vi "meTEC_Read_Firmware Indentification String.vi"(8 "error in (no error)":errorcluster, 9 "TEC Configuration_IN":T1={"VISA resource name"="", "Device Address"=2}, 11 "Sequence No.":u16=5546) -> (0 "error out":errorcluster, 1 "TEC Configuration_OUT":T1={"VISA resource name"="", "Device Address"=2}, 3 "Firmware Identification String":string)   [LabVIEW 2019]
uses:
  TypeDefs/meTEC_Configuration.ctl
panel:
  # "--- Inputs ---"
  # "--- Outputs ---"
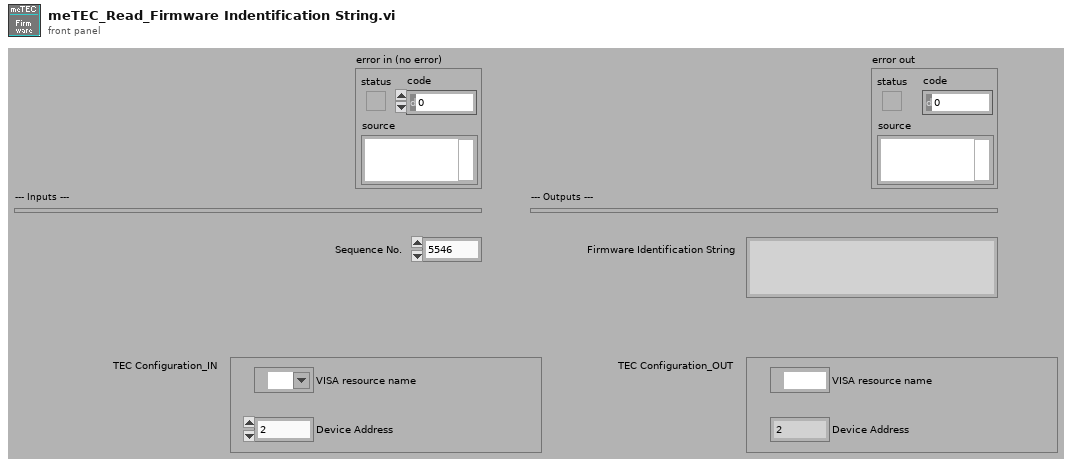
[diagram p1: front panel]
types:
  T1 = typedef "meTEC_Configuration.ctl" = cluster{"VISA resource name":refnum<visa-resource-name>, "Device Address":u16}
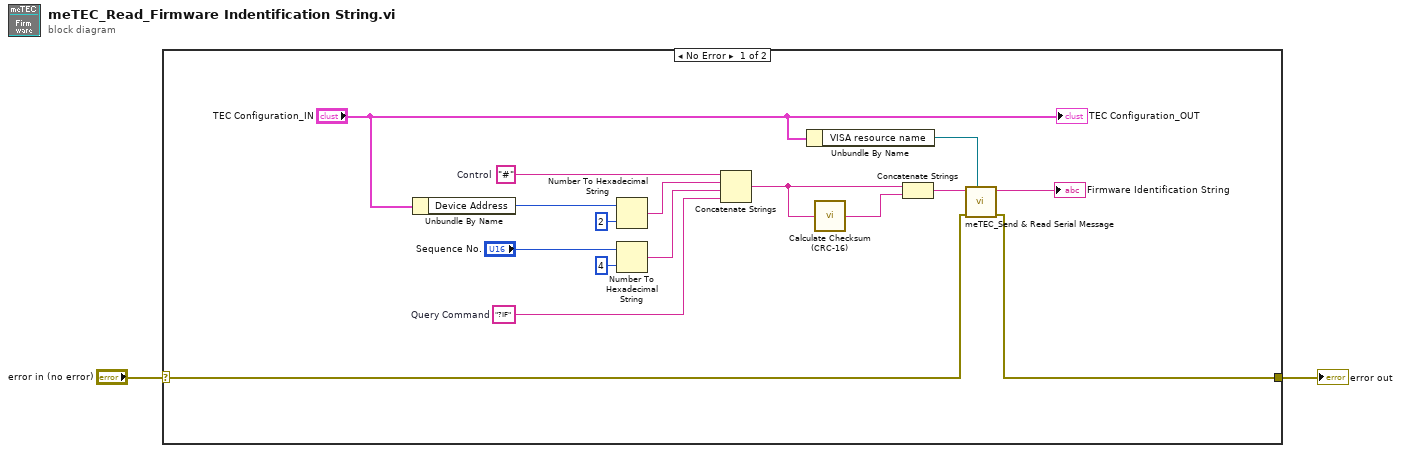
[diagram p0: block diagram]
diagram:
  n1 = case shown="No Error" "error in (no error)" {
    selector: "error in (no error)" -> [w7 w19]
    tunnel: [w6 w19] -> w2
    frame No Error {
      w16 = "#"  # Control
      w10 = "?IF"  # Query Command
      n2 = Unbundle By Name("TEC Configuration_IN") -> ("Device Address"=w3:u16)
      n3 = Number To Hexadecimal String(1:i16 2 ("width (-)"), 2:w3) -> (0:w11:string)
      n4 = Number To Hexadecimal String(1:i16 4 ("width (-)"), 2:"Sequence No.") -> (0:w15:string)
      n5 = Concatenate Strings(w16, w11, w15, w10) -> (w14:string)
      n6 = Unbundle By Name("TEC Configuration_IN") -> ("VISA resource name"=w5:refnum<visa-resource-name>)
      n7 = call "Calculate Checksum (CRC-16).vi"("Message"=w14) -> ("CRC [String]"=w13:string)  [unwired: 1 in]
      n8 = Concatenate Strings(w14, w13) -> (w8:string)
      n9 = call "meTEC_Send & Read Serial Message.vi"("VISA resource name"=w5, "error in (no error)"=w7, "Serial Message"=w8) -> ("error out"=w6:errorcluster, "Serial Message_Read"=→"Firmware Identification String":string)  [unwired: 7 in]
      "TEC Configuration_OUT" <- "TEC Configuration_IN"
    }
    frame Error {
    }
  }
  "error out" <- w2
